vi "Destroy_JQMHStartup.vi"(8 "error in (no error)":errorcluster, 11 "JQMHStartup in":refnum<class "RQMHStartup.lvclass">) -> (0 "error out":errorcluster)   [LabVIEW 2024, in "RQMHStartup.lvclass"]
uses:
  RQMHStartup.lvclass
  RQMHStartup.lvclass/RQMHStartup.ctl
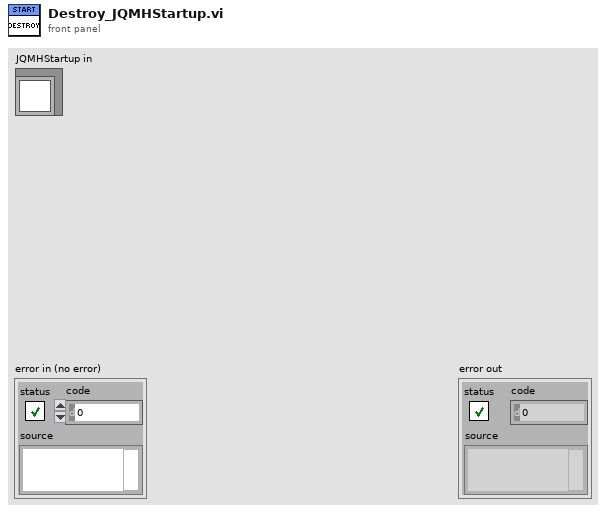
[diagram p1: front panel]
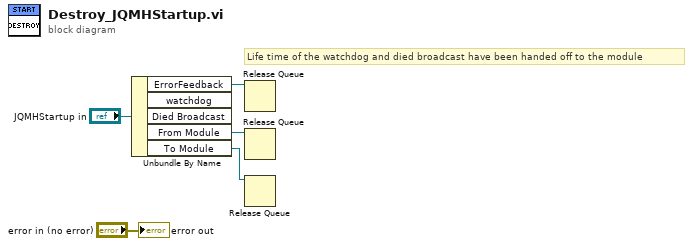
[diagram p0: block diagram]
diagram:
  # "Life time of the watchdog and died broadcast have been handed off to the module"
  n1 = Unbundle By Name("JQMHStartup in") -> ("ErrorFeedback"=w3:refnum<queue>, "From Module"=w2:refnum<queue>, "To Module"=w1:refnum<queue>)  [unwired: 2 out]
  n2 = Release Queue(queue=w3) -> ()  [unwired: 2 in, 3 out]
  n3 = Release Queue(queue=w2) -> ()  [unwired: 2 in, 3 out]
  n4 = Release Queue(queue=w1) -> ()  [unwired: 2 in, 3 out]
  "error out" <- "error in (no error)"
